vi "motor_controller.vi"() -> ()   [LabVIEW 2015]
uses:
  <vilib>/Analysis/baseanly.llb/Mean (DBL).vi
  <vilib>/Analysis/NI_AALBase.lvlib
panel:
  out "Grapher VI":refnum<vi>
  out "Simulation VI":refnum<vi>
  in  "Make up fit parameters":bool
  in  "Automatic velocity (rev/sec)":dbl=0.1 min=0.0 max=1.0
  in  "Reseek":bool
  in  "Automatic step size (rev)":dbl=0.01 min=0.0 max=1.0
  in  "Refine fit parameters":bool
  out "Fit parameters":cluster{"Slope":dbl, "Intercept":dbl}
  in  "Calculate fit parameters":bool
  in  "Read position 2":bool
  in  "Read position 1":bool
  out "Position 2":dbl
  in  "Frequency 2":dbl=140.4 min=0.0 step=0.001 format="%.3g"
  out "Position 1":dbl
  in  "Frequency 1":dbl=140.0 min=0.0 step=0.001 format="%.3g"
  in  "Seek positive polarization":bool=TRUE
  in  "Launch simulation":bool
  out "Polarization":dbl
  out "Eventnum":i64
  out "Samples taken":i32
  out "Rate":dbl
  in  "Data input file":path
  in  "Automatic mode on/off":bool
  in  "Goto frequency":bool
  in  "Frequency to seek (GHz)":dbl format="%.3g"
  in  "Stop motor":bool
  in  "Move up":bool
  in  "Move down":bool
  in  "Velocity (rev/sec)":dbl min=0.0 max=1.0 step=0.001
  in  "Step size (rev)":dbl=0.01 min=0.0 max=5.0 step=0.001
  in  "Stop communication":bool
  in  "COM Port":refnum<visa-resource-name>
  out "Alarm":bool
  out "Alarm code":u32 format="0x%02x"
  out "Frequency (calculated, GHz)":dbl format="%.3g"
  out "Motor position (rev)":dbl
  out "Motor time (sec)":dbl
  # "Advanced configuration"
  # "Frequency calibration"
  # "Automatic control"
  # "Manual motor control"
  # "Communication setup"
  # "Please wait after stopping the VI; it can take some time to shut down all the stuff running in the background, so please be patient."
  # "Motor alarm (error)"
  # "See motor manual, section \"Troubleshooting\" for explanation of alarm codes; fix the problem first and then restart this VI"
  # "Motor information"
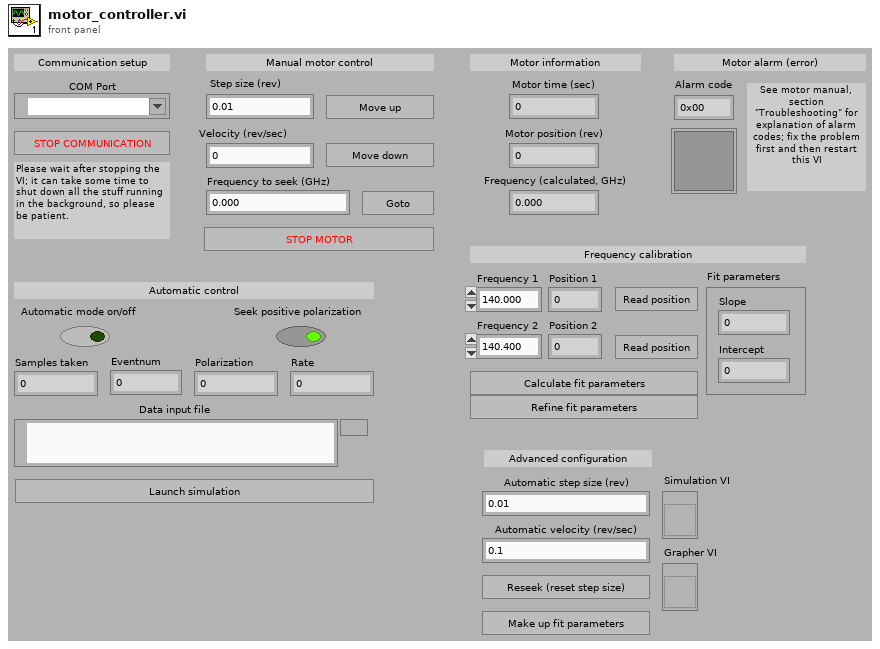
[diagram p1: front panel]
types:
  T1 = typedef "Semaphore RefNum" = refnum<k1>
  T2 = enum8{"Enabled", "Disabled", "Disabled and Grayed Out"}
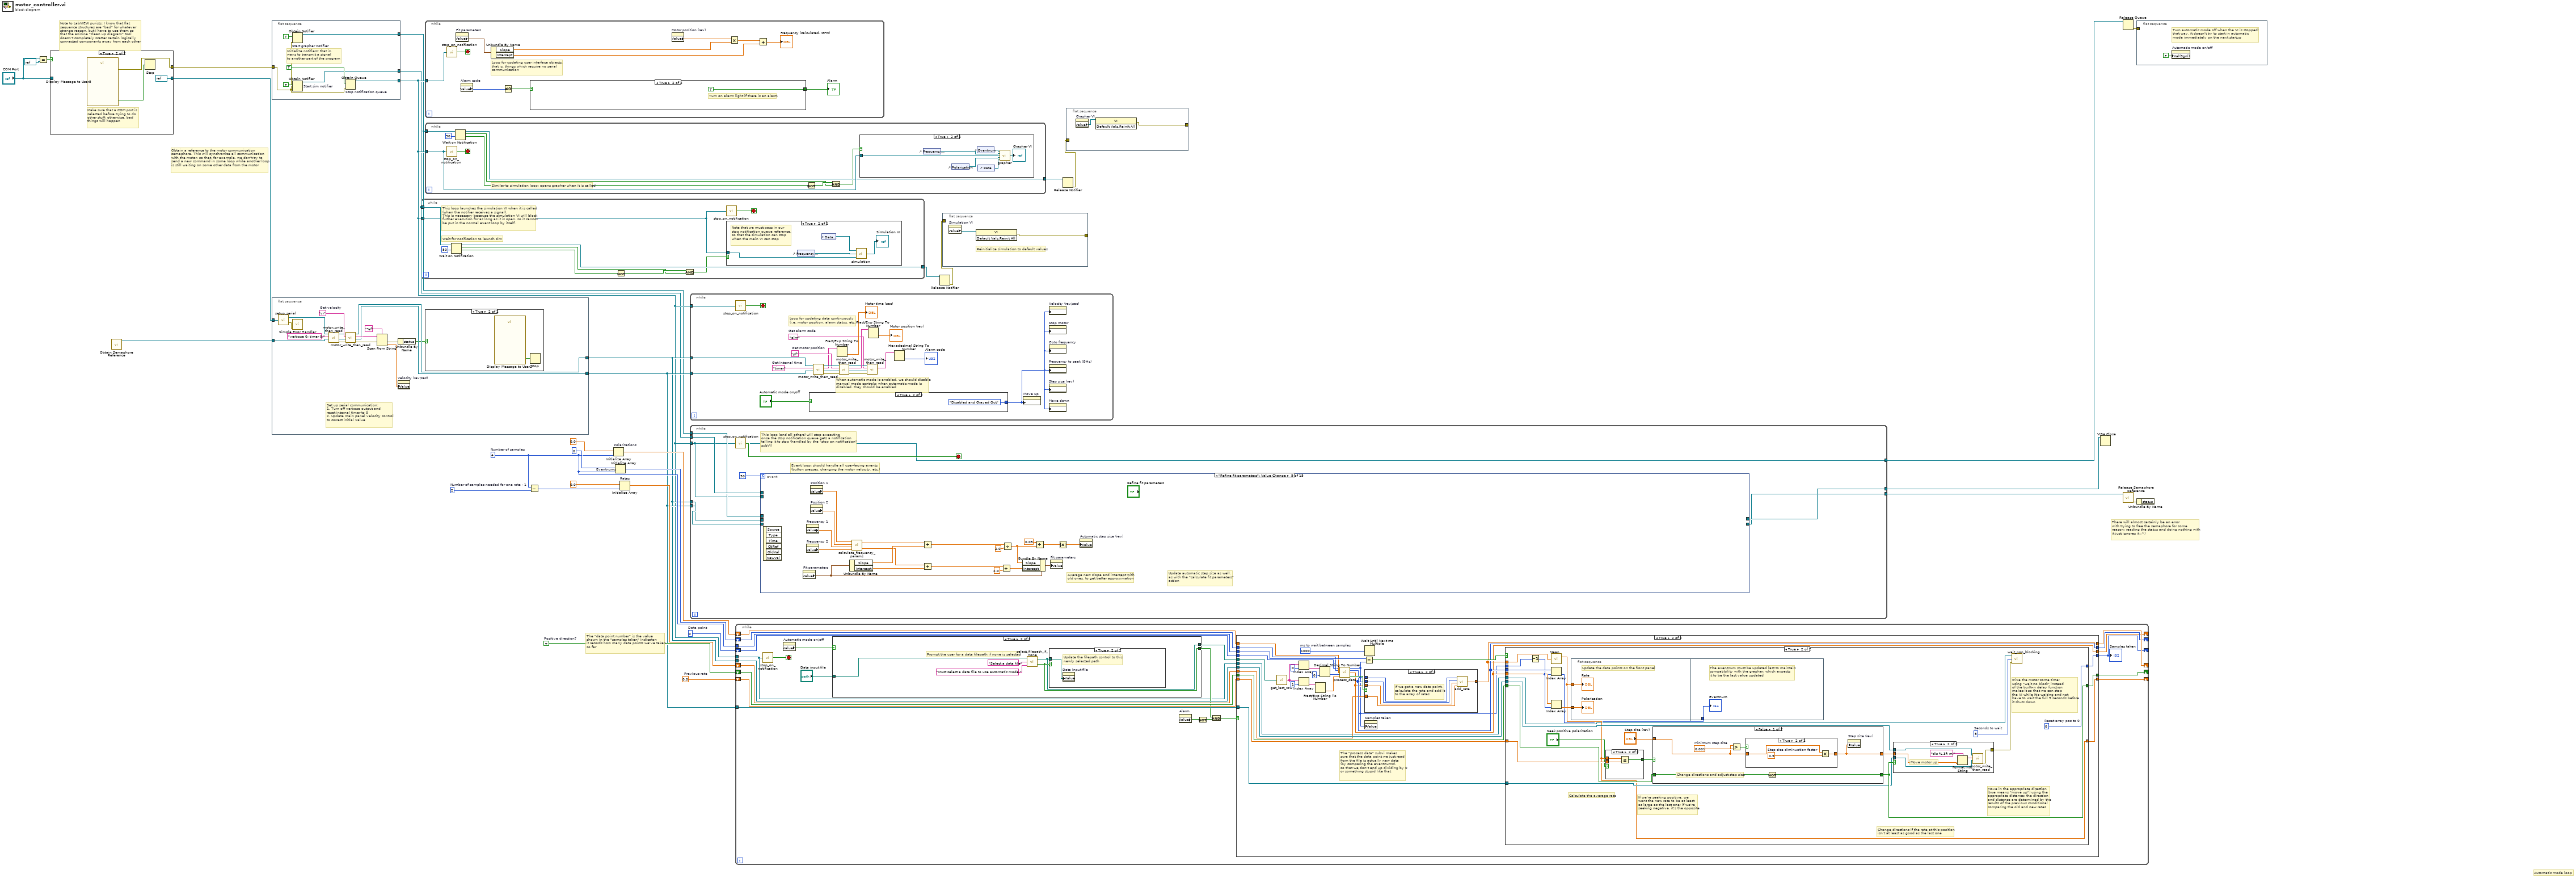
[diagram p0: block diagram]
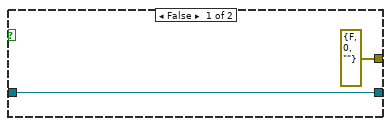
[diagram p4: hidden frame]
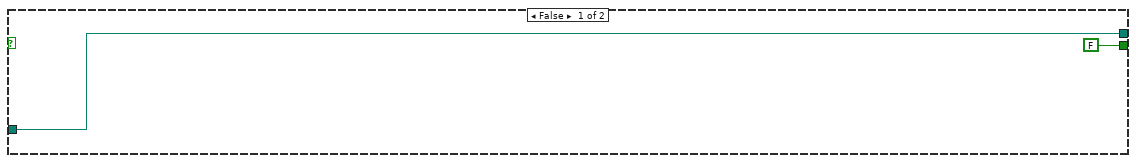
[diagram p6: hidden frame]
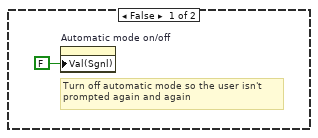
[diagram p7: hidden frame]
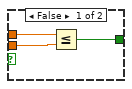
[diagram p11: hidden frame]
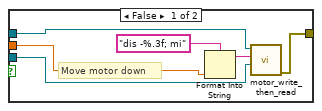
[diagram p12: hidden frame]
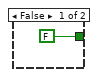
[diagram p15: hidden frame]
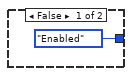
[diagram p16: hidden frame]
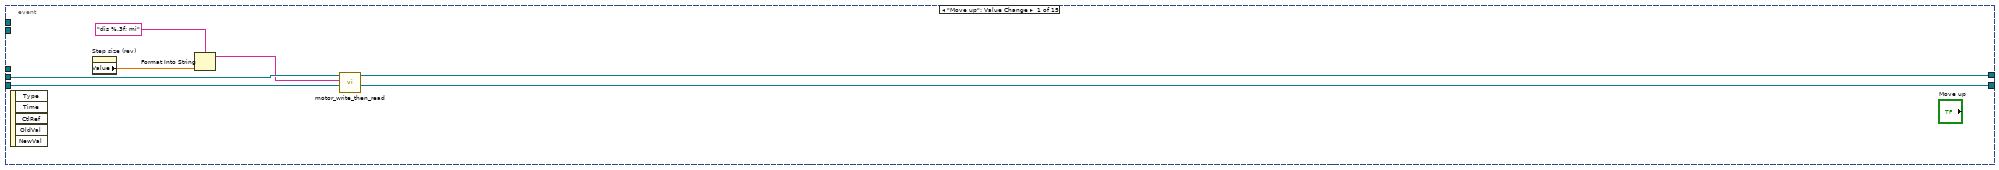
[diagram p17: hidden frame]
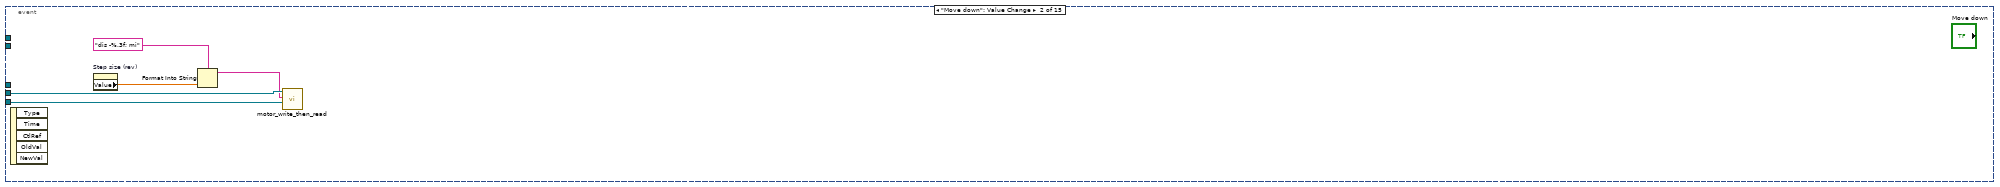
[diagram p18: hidden frame]
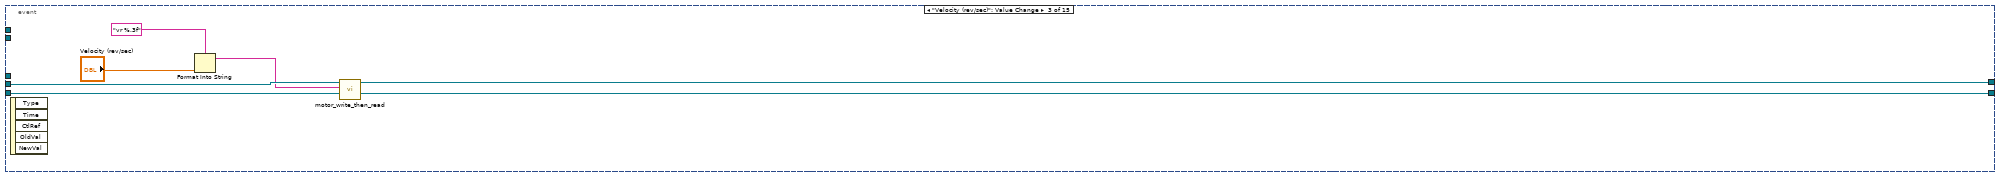
[diagram p19: hidden frame]
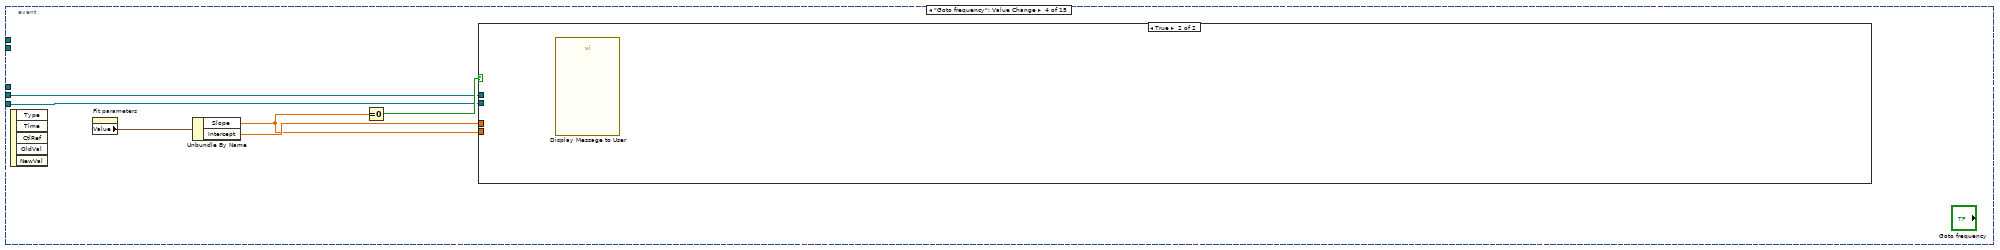
[diagram p20: hidden frame]
diagram:
  w17 = TRUE  # Positive direction?
  w18 = 0.0  # Previous rate
  w21 = 2  # Number of samples needed for one rate - 1
  w19 = 4  # Number of samples
  w28 = 0  # Data point
  # "There will almost certainly be an error\nwith trying to free the semaphore for some\nreason; reading the status and doing nothing with\nit just ignores it :^)"
  # "Obtain a reference to the motor communication\nsemaphore. This will synchronize all communication\nwith the motor, so that, for example, we don't try to\nsend a new command in some loop while another loop\nis still waiting on some other data from the motor"
  # "The \"data point number\" is the value\nshown in the \"samples taken\" indicator;\nit records how many data points we've taken\nso far"
  # "Automatic mode loop"
  # "Note to LabVIEW purists: I know that flat\nsequence structures are \"bad\" for whatever\nstrange reason, but I have to use them so\nthat the asinine \"clean up diagram\" tool\ndoesn't completely scatter certain logically\nconnected components away from each other"
  n1 = Equal?(x="COM Port", y=refnum<visa-resource-name> refnum) -> (x = y?=w12:bool)
  n2 = case shown="True" w12 {
    tunnel: "COM Port" -> [w34 _]
    tunnel: [w34 refnum<visa-resource-name> refnum ("COM Port")] -> w8
    tunnel: [errorcluster {"status"=FALSE, "code"=0, "source"=""} ("error out") w35] -> w3
    frame False {
    }
    frame True {
      # "Make sure that a COM port is\nselected before trying to do\nother stuff; otherwise, bad\nthings will happen"
      n3 = call "Display Message to User5"() -> ("error out"=w35:errorcluster, "I'm very sorry"=w36:bool)  [unwired: 10 in]
      n4 = Stop(stop? (T)=w36) -> ()
    }
  }
  n5 = call <vilib>:"Obtain Semaphore Reference.vi"() -> ("semaphore"=w7:T1)  [unwired: 5 in, 2 out]
  n6 = flat-sequence {
    tunnel: [w41] -> w6
    tunnel: [w40] -> w5
    tunnel: [w39] -> w4
    tunnel: w3 -> [w38]
    frame #0 {
      # "Initialize notifiers; that is,\nways to transmit a signal\nto another part of the program"
      n7 = Obtain Notifier "Start grapher notifier"(notification data type=TRUE, error in (no error)=w38) -> (notifier out=w40:refnum<notifier>)  [unwired: 2 in, 2 out]
      n8 = Obtain Notifier "Start sim notifier"(notification data type=TRUE, error in (no error)=w38) -> (notifier out=w39:refnum<notifier>)  [unwired: 2 in, 2 out]
      n9 = Obtain Queue "Stop notification queue"(element data type=TRUE, error in (no error)=w38) -> (queue out=w41:refnum<queue>)  [unwired: 3 in, 2 out]
    }
  }
  n10 = flat-sequence {
    tunnel: [w48] -> w10
    tunnel: [w49] -> w9
    tunnel: w8 -> [w50]
    tunnel: w7 -> [w47]
    frame #0 {
      w58 = "vr"  # Get velocity
      # "Set up serial communication:\n1. Turn off verbose output and\nreset internal timer to 0\n2. Update main panel velocity control\nto correct initial value"
      n11 = call "setup_serial.vi"("COM Port"=w50) -> ("error out"=w52:errorcluster, "VISA resource name out"=w55:refnum<visa-resource-name>)
      n12 = call <vilib>:"Simple Error Handler.vi"("error in (no error)"=w52) -> ()  [unwired: 4 in, 5 out]
      n13 = call "motor_write_then_read.vi"("Semaphore in"=w47, "Data to write"="verbose 0; timer 0;", "VISA resource name in"=w55) -> ("Error out"=w61:errorcluster, "Semaphore out"=w51:T1, "VISA resource name out"=w57:refnum<visa-resource-name>)  [unwired: 1 in, 1 out]
      n14 = call "motor_write_then_read.vi"("Error in"=w61, "Semaphore in"=w51, "Data to write"=w58, "VISA resource name in"=w57) -> ("Error out"=w60:errorcluster, "Semaphore out"=w48:T1, "Received data"=w59:string, "VISA resource name out"=w49:refnum<visa-resource-name>)
      n15 = Scan From String(format string="%f", input string=w59, error in=w60) -> (error out=w46:errorcluster, output 1=w54:dbl)  [unwired: 2 in, 2 out]
      n16 = Unbundle By Name(w46) -> ("status"=w45:bool)
      n17 = property on="Velocity (rev/sec)" class="DigNum (strict)"("Value"=w54) -> ()  [unwired: 2 in, 2 out]
      n18 = case shown="True" w45 {
        frame False {
        }
        frame True {
          n19 = call "Display Message to User2"() -> ("Thanks, I'll try that"=w62:bool)  [unwired: 10 in, 1 out]
          n20 = Stop(stop? (T)=w62) -> ()
        }
      }
    }
  }
  n21 = while {
    tunnel: w6 -> [w63]
    tunnel: w4 -> [w69]
    tunnel: [w68] -> w15
    stop <- w71 stop-if-true
    # "This loop launches the simulation VI when it is called\n(when the notifier receives a signal).\nThis is necessary because the simulation VI will block\nfurther execution for as long as it is open, so it cannot\nbe put in the normal event loop by itself."
    # "Wait for notification to launch sim"
    n22 = Wait on Notification(notifier=w69, timeout in ms (-1)=50) -> (notifier out=w68:refnum<notifier>, notification=w65:bool, timed out?=w66:bool)  [unwired: 2 in, 1 out]
    n23 = Not(x=w66) -> (.not. x?=w67:bool)
    n24 = And(x=w67, y=w65) -> (x .and. y?=w64:bool)
    n25 = call "stop_on_notification.vi"("Notofication queue"=w63) -> ("Should stop"=w71:bool)
    n26 = case shown="True" w64 {
      tunnel: w63 -> [_ w75]
      frame False {
      }
      frame True {
        # "Note that we must pass in our\nstop notification queue reference,\nso that the simulation can stop\nwhen the main VI can stop"
        n27 = control-ref of="Frequency (calculated, GHz)"() -> (w74:refnum<vi>)
        n28 = control-ref of="Data input file"() -> (w73:refnum<vi>)
        n29 = call "simulation.vi"("Stop notification queue"=w75, "Frequency refnum"=w74, "Filepath refnum"=w73) -> ("This VI refnum"=→"Simulation VI":refnum<vi>)
      }
    }
  }
  n30 = while {
    tunnel: w6 -> [w79]
    stop <- w78 stop-if-true
    # "Loop for updating user interface objects,\nthat is, things which require no serial\ncommunication"
    n31 = call "stop_on_notification.vi"("Notofication queue"=w79) -> ("Should stop"=w78:bool)
    n32 = property on="Fit parameters" class="Clust (strict)"() -> ("Value"=w85:cluster{"Slope":dbl, "Intercept":dbl})  [unwired: 2 in, 2 out]
    n33 = property on="Alarm code" class="DigNum (strict)"() -> ("Value"=w77:u32)  [unwired: 2 in, 2 out]
    n34 = Unbundle By Name(w85) -> ("Slope"=w83:dbl, "Intercept"=w80:dbl)
    n35 = Not Equal To 0?(x=w77) -> (x != 0?=w76:bool)
    n36 = case shown="True" w76 {
      tunnel: [FALSE TRUE] -> w86
      frame False {
      }
      frame True {
        # "Turn on alarm light if there is an alarm"
      }
    }
    "Alarm" <- w86
    n37 = property on="Motor position (rev)" class="DigNum (strict)"() -> ("Value"=w84:dbl)  [unwired: 2 in, 2 out]
    n38 = Multiply(x=w84, y=w83) -> (x*y=w81:dbl)
    n39 = Add(x=w81, y=w80) -> (x+y=→"Frequency (calculated, GHz)":dbl)
  }
  n40 = while {
    tunnel: w6 -> [w96]
    tunnel: w5 -> [w94]
    tunnel: [w93] -> w11
    stop <- w97 stop-if-true
    # "Similar to simulation loop; opens grapher when it is called"
    n41 = call "stop_on_notification.vi"("Notofication queue"=w96) -> ("Should stop"=w97:bool)
    n42 = Wait on Notification(notifier=w94, timeout in ms (-1)=50) -> (notifier out=w93:refnum<notifier>, notification=w91:bool, timed out?=w90:bool)  [unwired: 2 in, 1 out]
    n43 = Not(x=w90) -> (.not. x?=w92:bool)
    n44 = And(x=w92, y=w91) -> (x .and. y?=w89:bool)
    n45 = case shown="True" w89 {
      tunnel: w96 -> [_ w100]
      frame False {
      }
      frame True {
        n46 = control-ref of="Frequency (calculated, GHz)"() -> (w101:refnum<vi>)
        n47 = control-ref of="Polarization"() -> (w102:refnum<vi>)
        n48 = control-ref of="Eventnum"() -> (w99:refnum<vi>)
        n49 = control-ref of="Rate"() -> (w103:refnum<vi>)
        n50 = call "grapher.vi"("Eventnum refnum"=w99, "Frequency refnum"=w101, "Stop notification queue"=w100, "Polarization refnum"=w102, "Rate refnum"=w103) -> ("This VI refnum"=→"Grapher VI":refnum<vi>)  [unwired: 10 in]
      }
    }
  }
  n51 = Subtract(x=w19, y=w21) -> (x-y=w22:i32)
  n52 = Initialize Array "Polarizations"(0.0, w19) -> (w25:dbl[])
  n53 = Initialize Array "Eventnums"(i64 0, w19) -> (w26:i64[])
  n54 = Initialize Array "Rates"(0.0 ("element"), w22) -> (w20:dbl[])
  n55 = while {
    tunnel: w10 -> [w123]
    tunnel: w9 -> [w124]
    tunnel: w6 -> [w106]
    stop <- w105 stop-if-true
    w110 = "alm"  # Get alarm code
    w118 = "pf"  # Get motor position
    w122 = "timer"  # Get internal time
    # "When automatic mode is enabled, we should disable\nmanual mode controls; when automatic mode is\ndisabled, they should be enabled"
    # "Loop for updating data continuously\n(i.e. motor position, alarm status, etc.)"
    n56 = call "stop_on_notification.vi"("Notofication queue"=w106) -> ("Should stop"=w105:bool)
    n57 = case shown="True" "Automatic mode on/off" {
      tunnel: [T2."Enabled" ("Disabled") T2."Disabled and Grayed Out" ("Disabled")] -> w104
      frame False {
      }
      frame True {
      }
    }
    n58 = call "motor_write_then_read.vi"("Semaphore in"=w123, "Data to write"=w122, "VISA resource name in"=w124) -> ("Error out"=w119:errorcluster, "Semaphore out"=w120:T1, "Received data"=w117:string, "VISA resource name out"=w121:refnum<visa-resource-name>)  [unwired: 1 in]
    n59 = Fract/Exp String To Number(string=w117) -> (number=→"Motor time (sec)":dbl)  [unwired: 3 in, 1 out]
    n60 = call "motor_write_then_read.vi"("Error in"=w119, "Semaphore in"=w120, "Data to write"=w118, "VISA resource name in"=w121) -> ("Error out"=w112:errorcluster, "Semaphore out"=w111:T1, "Received data"=w115:string, "VISA resource name out"=w113:refnum<visa-resource-name>)
    n61 = call "motor_write_then_read.vi"("Error in"=w112, "Semaphore in"=w111, "Data to write"=w110, "VISA resource name in"=w113) -> ("Received data"=w109:string)  [unwired: 3 out]
    n62 = Fract/Exp String To Number(string=w115) -> (number=→"Motor position (rev)":dbl)  [unwired: 3 in, 1 out]
    n63 = Hexadecimal String To Number(string=w109) -> (number=→"Alarm code":u32)  [unwired: 2 in, 1 out]
    n64 = property on="Move up" class="Bool"("DisabledEnum"=w104) -> ()  [unwired: 2 in, 2 out]
    n65 = property on="Velocity (rev/sec)" class="DigNum (strict)"("DisabledEnum"=w104) -> ()  [unwired: 2 in, 2 out]
    n66 = property on="Stop motor" class="Bool"("DisabledEnum"=w104) -> ()  [unwired: 2 in, 2 out]
    n67 = property on="Goto frequency" class="Bool"("DisabledEnum"=w104) -> ()  [unwired: 2 in, 2 out]
    n68 = property on="Frequency to seek (GHz)" class="DigNum (strict)"("DisabledEnum"=w104) -> ()  [unwired: 2 in, 2 out]
    n69 = property on="Step size (rev)" class="DigNum (strict)"("DisabledEnum"=w104) -> ()  [unwired: 2 in, 2 out]
    n70 = property on="Move down" class="Bool"("DisabledEnum"=w104) -> ()  [unwired: 2 in, 2 out]
  }
  n71 = while {
    tunnel: w10 -> [w135]
    tunnel: w9 -> [w134]
    tunnel: [w133] -> w32
    tunnel: [w132] -> w31
    tunnel: w6 -> [w127]
    tunnel: [w127] -> w29
    tunnel: w4 -> [w131]
    tunnel: w5 -> [w130]
    stop <- w129 stop-if-true
    # "This loop (and all others) will stop executing\nonce the stop notification queue gets a notification\ntelling it to stop (handled by the \"stop on notification\"\nsubVI)"
    # "Event loop; should handle all user-facing events\n(button presses, changing the motor velocity, etc.)"
    n72 = call "stop_on_notification.vi"("Notofication queue"=w127) -> ("Should stop"=w129:bool)
    n73 = event shown="[8] \"Refine fit parameters\": Value Change" {
      selector: _ -> [_ _ _ _ _ _ _ _ _ _ _ _ _ _ _]
      dyn-events: _ -> [_ _ _ _ _ _ _ _ _ _ _ _ _ _ _]
      timeout: 50 -> [_ _ _ _ _ _ _ _ _ _ _ _ _ _ _]
      tunnel: w135 -> [w139 w143 w150 w155 w186 _ _ _ _ _ _ _ _ _ w250]
      tunnel: w134 -> [w140 w145 w152 w156 w192 _ _ _ _ _ _ _ _ _ w251]
      tunnel: [w138 _ w148 _ _ _ _ _ _ _ _ _ _ _ w251] -> w133
      tunnel: [w137 _ w149 _ _ _ _ _ _ _ _ _ _ _ w250] -> w132
      tunnel: w131 -> [_ _ _ _ _ _ _ _ _ w228 _ _ _ _ _]
      tunnel: w130 -> [_ _ _ _ _ _ _ _ _ _ _ w236 _ _ _]
      tunnel: w127 -> [_ _ _ _ _ _ _ _ _ _ _ _ _ w248 _]
      event "Move up": Value Change {
        n74 = event-data() -> ()  [unwired: 1 in, 5 out]
        n75 = property on="Step size (rev)" class="DigNum (strict)"() -> ("Value"=w141:dbl)  [unwired: 2 in, 2 out]
        n76 = Format Into String(format string="dis %.3f; mi", w141) -> (resulting string=w136:string)  [unwired: 2 in, 1 out]
        n77 = call "motor_write_then_read.vi"("Semaphore in"=w139, "Data to write"=w136, "VISA resource name in"=w140) -> ("Semaphore out"=w137:T1, "VISA resource name out"=w138:refnum<visa-resource-name>)  [unwired: 1 in, 2 out]
      }
      event "Move down": Value Change {
        n78 = event-data() -> ()  [unwired: 1 in, 5 out]
        n79 = property on="Step size (rev)" class="DigNum (strict)"() -> ("Value"=w146:dbl)  [unwired: 2 in, 2 out]
        n80 = Format Into String(format string="dis -%.3f; mi", w146) -> (resulting string=w144:string)  [unwired: 2 in, 1 out]
        n81 = call "motor_write_then_read.vi"("Semaphore in"=w143, "Data to write"=w144, "VISA resource name in"=w145) -> ()  [unwired: 1 in, 4 out]
      }
      event "Velocity (rev/sec)": Value Change {
        n82 = event-data() -> ()  [unwired: 1 in, 5 out]
        n83 = Format Into String(format string="vr %.3f", "Velocity (rev/sec)") -> (resulting string=w151:string)  [unwired: 2 in, 1 out]
        n84 = call "motor_write_then_read.vi"("Semaphore in"=w150, "Data to write"=w151, "VISA resource name in"=w152) -> ("Semaphore out"=w149:T1, "VISA resource name out"=w148:refnum<visa-resource-name>)  [unwired: 1 in, 2 out]
      }
      event "Goto frequency": Value Change {
        n85 = event-data() -> ()  [unwired: 1 in, 5 out]
        n86 = property on="Fit parameters" class="Clust (strict)"() -> ("Value"=w160:cluster{"Slope":dbl, "Intercept":dbl})  [unwired: 2 in, 2 out]
        n87 = Unbundle By Name(w160) -> ("Slope"=w157:dbl, "Intercept"=w158:dbl)
        n88 = Equal To 0?(x=w157) -> (x = 0?=w159:bool)
        n89 = case shown="True" w159 {
          tunnel: w158 -> [w173 _]
          tunnel: w157 -> [w171 _]
          tunnel: w156 -> [w168 _]
          tunnel: w155 -> [w167 _]
          frame False {
            # "Calculate corresponding motor position and go there"
            n90 = Subtract(x="Frequency to seek (GHz)", y=w173) -> (x-y=w172:dbl)
            n91 = property on="Motor position (rev)" class="DigNum (strict)"() -> ("Value"=w169:dbl)  [unwired: 2 in, 2 out]
            n92 = Divide(x=w172, y=w171) -> (x/y=w170:dbl)
            n93 = Subtract(x=w170, y=w169) -> (x-y=w165:dbl)
            n94 = Absolute Value(x=w165) -> (abs(x)=w164:dbl)
            n95 = Less?(x=w164, y=1.0) -> (x < y?=w161:bool)
            n96 = case shown="False" w161 {
              selector: w161 -> [_ w178]
              tunnel: [w174 w178] -> w162
              frame False {
                n97 = Two Button Dialog(message="The frequency you are attempting to go to is very far from the current position; you may run into problems. Are you sure you want to continue?", 1:"No" ("F button name (\"Cancel\")"), 2:"Yes" ("T button name (\"OK\")")) -> (T button?=w174:bool)
              }
              frame True {
              }
            }
            n98 = case shown="True" w162 {
              tunnel: w168 -> [_ w183]
              tunnel: w165 -> [_ w182]
              tunnel: w167 -> [_ w179]
              frame False {
              }
              frame True {
                n99 = Format Into String(format string="dis %.3f; mi", w182) -> (resulting string=w180:string)  [unwired: 2 in, 1 out]
                n100 = call "motor_write_then_read.vi"("Semaphore in"=w179, "Data to write"=w180, "VISA resource name in"=w183) -> ()  [unwired: 1 in, 4 out]
              }
            }
          }
          frame True {
            n101 = call "Display Message to User"() -> ()  [unwired: 10 in, 2 out]
          }
        }
      }
      event "Stop motor": Value Change {
        n102 = event-data() -> ()  [unwired: 1 in, 5 out]
        n103 = call <vilib>:"Acquire Semaphore.vi"("semaphore"=w186) -> ("error out"=w190:errorcluster, "semaphore out"=w185:T1)  [unwired: 4 in, 1 out]
        n104 = VISA Write(VISA resource name=w192, write buffer="mstop\r", error in (no error)=w190) -> (VISA resource name out=w194:refnum<visa-resource-name>, error out=w189:errorcluster)  [unwired: 1 out]
        n105 = VISA Read(VISA resource name=w194, byte count=u32 1, error in (no error)=w189) -> (VISA resource name out=w193:refnum<visa-resource-name>, error out=w188:errorcluster)  [unwired: 2 out]
        n106 = VISA Flush I/O Buffer(VISA resource name=w193, error in (no error)=w188) -> (error out=w187:errorcluster)  [unwired: 1 in, 1 out]
        n107 = call <vilib>:"Release Semaphore.vi"("error in (no error)"=w187, "semaphore"=w185) -> ()  [unwired: 4 in, 2 out]
      }
      event "Read position 1": Value Change {
        n108 = event-data() -> ()  [unwired: 1 in, 5 out]
        n109 = property on="Motor position (rev)" class="DigNum (strict)"() -> ("Value"=→"Position 1":dbl)  [unwired: 2 in, 2 out]
      }
      event "Read position 2": Value Change {
        n110 = event-data() -> ()  [unwired: 1 in, 5 out]
        n111 = property on="Motor position (rev)" class="DigNum (strict)"() -> ("Value"=→"Position 2":dbl)  [unwired: 2 in, 2 out]
      }
      event "Calculate fit parameters": Value Change {
        # "The automatic step size should be around 0.05GHz\ninitially, to get a good seek"
        # "Calculate slope and intercept"
        n112 = event-data() -> ()  [unwired: 1 in, 5 out]
        n113 = property on="Position 1" class="DigNum (strict)"() -> ("Value"=w205:dbl)  [unwired: 2 in, 2 out]
        n114 = property on="Position 2" class="DigNum (strict)"() -> ("Value"=w204:dbl)  [unwired: 2 in, 2 out]
        n115 = property on="Calculate fit parameters" class="Bool (strict)"("Value"=FALSE ("Calculate fit parameters")) -> ()  [unwired: 2 in, 2 out]
        n116 = call "calculate_frequency_params.vi"("Frequency 2"="Frequency 2", "Frequency 1"="Frequency 1", "Position 2"=w204, "Position 1"=w205) -> ("Intercept"=w206:dbl, "Slope"=w199:dbl)
        n117 = Divide(x=0.05, y=w199) -> (x/y=w198:dbl)
        n118 = property on="Fit parameters" class="Clust (strict)"() -> ("Value"=w208:cluster{"Slope":dbl, "Intercept":dbl})  [unwired: 2 in, 2 out]
        n119 = Bundle By Name(cluster=w208, "Slope"=w199, "Intercept"=w206) -> (→"Fit parameters":cluster{"Slope":dbl, "Intercept":dbl})
        n120 = Absolute Value(x=w198) -> (abs(x)=w197:dbl)
        n121 = property on="Automatic step size (rev)" class="DigNum (strict)"("Value"=w197) -> ()  [unwired: 2 in, 2 out]
      }
      event "Refine fit parameters": Value Change {
        # "Update automatic step size as well,\nas with the \"calculate fit parameters\"\naction"
        # "Average new slope and intercept with\nold ones, to get better approximation"
        n122 = event-data() -> ()  [unwired: 1 in, 6 out]
        n123 = property on="Fit parameters" class="Clust (strict)"() -> ("Value"=w214:cluster{"Slope":dbl, "Intercept":dbl})  [unwired: 2 in, 2 out]
        n124 = property on="Frequency 1" class="DigNum (strict)"() -> ("Value"=w227:dbl)  [unwired: 2 in, 2 out]
        n125 = property on="Frequency 2" class="DigNum (strict)"() -> ("Value"=w226:dbl)  [unwired: 2 in, 2 out]
        n126 = property on="Position 1" class="DigNum (strict)"() -> ("Value"=w225:dbl)  [unwired: 2 in, 2 out]
        n127 = property on="Position 2" class="DigNum (strict)"() -> ("Value"=w224:dbl)  [unwired: 2 in, 2 out]
        n128 = Unbundle By Name(w214) -> ("Slope"=w222:dbl, "Intercept"=w220:dbl)
        n129 = call "calculate_frequency_params.vi"("Frequency 2"=w226, "Frequency 1"=w227, "Position 2"=w224, "Position 1"=w225) -> ("Intercept"=w221:dbl, "Slope"=w223:dbl)
        n130 = Add(x=w223, y=w222) -> (x+y=w219:dbl)
        n131 = Add(x=w221, y=w220) -> (x+y=w218:dbl)
        n132 = Divide(x=w218, y=2.0) -> (x/y=w213:dbl)
        n133 = Divide(x=w219, y=2.0) -> (x/y=w211:dbl)
        n134 = Bundle By Name(cluster=w214, "Slope"=w211, "Intercept"=w213) -> (w215:cluster{"Slope":dbl, "Intercept":dbl})
        n135 = Divide(x=0.05, y=w211) -> (x/y=w210:dbl)
        n136 = property on="Fit parameters" class="Clust (strict)"("Value"=w215) -> ()  [unwired: 2 in, 2 out]
        n137 = Absolute Value(x=w210) -> (abs(x)=w209:dbl)
        n138 = property on="Automatic step size (rev)" class="DigNum (strict)"("Value"=w209) -> ()  [unwired: 2 in, 2 out]
      }
      event "Launch simulation": Value Change {
        # "Tell the simulation notifier to launch the simulation"
        n139 = event-data() -> ()  [unwired: 1 in, 5 out]
        n140 = property on="Fit parameters" class="Clust (strict)"() -> ("Value"=w231:cluster{"Slope":dbl, "Intercept":dbl})  [unwired: 2 in, 2 out]
        n141 = Unbundle By Name(w231) -> ("Slope"=w230:dbl)
        n142 = Equal To 0?(x=w230) -> (x = 0?=w229:bool)
        n143 = case shown="True" w229 {
          tunnel: w228 -> [w232 _]
          frame False {
            n144 = Send Notification(notification=TRUE, notifier=w232) -> ()  [unwired: 1 in, 2 out]
          }
          frame True {
            n145 = call "Display Message to User3"() -> ()  [unwired: 10 in, 2 out]
          }
        }
      }
      event "Reseek": Value Change {
        # "Change step size back to the default (initial) automatic step size"
        n146 = event-data() -> ()  [unwired: 1 in, 5 out]
        n147 = property on="Automatic mode on/off" class="Bool (strict)"() -> ("Value"=w234:bool)  [unwired: 2 in, 2 out]
        n148 = case shown="True" w234 {
          frame False {
          }
          frame True {
            n149 = property on="Automatic step size (rev)" class="DigNum (strict)"() -> ("Value"=w235:dbl)  [unwired: 2 in, 2 out]
            n150 = property on="Step size (rev)" class="DigNum (strict)"("Value"=w235) -> ()  [unwired: 2 in, 2 out]
          }
        }
      }
      event "Automatic mode on/off": Value Change {
        # "When automatic mode is first enabled,\nchoose the initial step size and start\ngrapher subvi"
        n151 = event-data() -> ()  [unwired: 1 in, 5 out]
        n152 = property on="Automatic mode on/off" class="Bool (strict)"() -> ("Value"=w237:bool)  [unwired: 2 in, 2 out]
        n153 = case shown="True" w237 {
          tunnel: w236 -> [_ w240]
          frame False {
          }
          frame True {
            n154 = Send Notification(notification=TRUE, notifier=w240) -> ()  [unwired: 1 in, 2 out]
            n155 = property on="Velocity (rev/sec)" class="DigNum (strict)"("Val(Sgnl)"="Automatic velocity (rev/sec)") -> ()  [unwired: 2 in, 2 out]
            n156 = property on="Step size (rev)" class="DigNum (strict)"("Val(Sgnl)"="Automatic step size (rev)") -> ()  [unwired: 2 in, 2 out]
          }
        }
      }
      event "Make up fit parameters": Value Change {
        # "Make up some fit parameters (no physical meaning)\nfor quick testing of automatic mode"
        n157 = event-data() -> ()  [unwired: 1 in, 5 out]
        n158 = flat-sequence {
          frame #0 {
            n159 = property on="Frequency 2" class="DigNum (strict)"("Value"=140.15 ("Frequency 2")) -> ()  [unwired: 2 in, 2 out]
            n160 = property on="Frequency 1" class="DigNum (strict)"("Value"=140.1 ("Frequency 1")) -> ()  [unwired: 2 in, 2 out]
            n161 = property on="Motor position (rev)" class="DigNum (strict)"() -> ("Value"=w246:dbl)  [unwired: 2 in, 2 out]
            n162 = property on="Position 2" class="DigNum (strict)"("Value"=w246) -> ()  [unwired: 2 in, 2 out]
            n163 = property on="Step size (rev)" class="DigNum (strict)"() -> ("Value"=w244:dbl)  [unwired: 2 in, 2 out]
            n164 = Subtract(x=w246, y=w244) -> (x-y=w245:dbl)
            n165 = property on="Position 1" class="DigNum (strict)"("Value"=w245) -> ()  [unwired: 2 in, 2 out]
          }
          frame #1 {
            n166 = property on="Calculate fit parameters" class="Bool (strict)"("Val(Sgnl)"=TRUE ("Value (Signaling)")) -> ()  [unwired: 2 in, 2 out]
          }
        }
      }
      event "Stop communication": Value Change {
        n167 = event-data() -> ()  [unwired: 1 in, 5 out]
        n168 = call "send_notification.vi"("Notification"="Stop communication", "Notification queue in"=w248) -> ()  [unwired: 1 out]
      }
      event Timeout {
        n169 = event-data() -> ()  [unwired: 1 in, 2 out]
      }
    }
  }
  n170 = while {
    tunnel: w6 -> [w252]
    shift-right: [w261] -> _
    shift-left: w28 -> [w257]
    shift-right: [w260] -> _
    shift-left: w26 -> [w271]
    shift-right: [w259] -> _
    shift-left: w25 -> [w270]
    shift-right: [w269] -> _
    shift-left: w20 -> [w262]
    tunnel: w19 -> [w268]
    shift-right: [w258] -> _
    shift-left: w18 -> [w267]
    shift-right: [w265] -> _
    shift-left: w17 -> [w266]
    tunnel: w9 -> [w264]
    tunnel: w10 -> [w263]
    stop <- w275 stop-if-true
    n171 = call "stop_on_notification.vi"("Notofication queue"=w252) -> ("Should stop"=w275:bool)
    n172 = property on="Automatic mode on/off" class="Bool (strict)"() -> ("Value"=w256:bool)  [unwired: 2 in, 2 out]
    n173 = case shown="True" w256 {
      tunnel: "Data input file" -> [w277 w280]
      tunnel: [w277 w278] -> w254
      tunnel: [FALSE ("Filepath valid?") w279] -> w253
      frame False {
      }
      frame True {
        # "Prompt the user for a data filepath if none is selected"
        n174 = call "select_filepath_if_none.vi"("Error message"="Must select a data file to use automatic mode.", "Selector prompt"="Select a data file", "Filepath in"=w280) -> ("Filepath valid?"=w279:bool, "Filepath out"=w278:path)
        n175 = case shown="True" w279 {
          tunnel: w278 -> [_ w284]
          frame False {
            # "Turn off automatic mode so the user isn't\nprompted again and again"
            n176 = property on="Automatic mode on/off" class="Bool (strict)"("Val(Sgnl)"=FALSE ("Value (Signaling)")) -> ()  [unwired: 2 in, 2 out]
          }
          frame True {
            # "Update the filepath control to this\nnewly selected path"
            n177 = property on="Data input file" class="Path"("Value"=w284) -> ()  [unwired: 2 in, 2 out]
          }
        }
      }
    }
    n178 = property on="Alarm" class="Bool (strict)"() -> ("Value"=w274:bool)  [unwired: 2 in, 2 out]
    n179 = Not(x=w274) -> (.not. x?=w273:bool)
    n180 = And(x=w253, y=w273) -> (x .and. y?=w272:bool)
    n181 = case shown="True" w272 {
      tunnel: w257 -> [w290 w294]
      tunnel: w271 -> [w289 w300]
      tunnel: w270 -> [w288 w301]
      tunnel: [w290 w313] -> w261
      tunnel: [w289 w298] -> w260
      tunnel: [w288 w297] -> w259
      tunnel: w262 -> [w287 w296]
      tunnel: [w287 w295] -> w269
      tunnel: w268 -> [_ w315]
      tunnel: [w286 w312] -> w258
      tunnel: w267 -> [w286 w311]
      tunnel: w266 -> [w285 w310]
      tunnel: [w285 w309] -> w265
      tunnel: w264 -> [_ w308]
      tunnel: w263 -> [_ w307]
      tunnel: w254 -> [_ w304]
      tunnel: w252 -> [_ w292]
      frame False {
      }
      frame True {
        w305 = u32 1000  # ms to wait between samples
        # "The \"process data\" subvi makes\nsure that the data point we just read\nfrom the file is actually new data\n(by comparing the eventnums),\nso that we don't end up dividing by 0\nor something stupid like that"
        n182 = call "get_last_row.vi"("Data input file"=w304) -> ("last row"=w306:string[])
        n183 = Index Array(array=w306, index=0) -> (element=w317:string)
        n184 = Index Array(array=w306, index=1) -> (element=w316:string)
        n185 = Fract/Exp String To Number(string=w316) -> (number=w302:dbl)  [unwired: 3 in, 1 out]
        n186 = Decimal String To Number(string=w317, default (0L)=i64 0 ("default (0 I32)")) -> (number=w303:i64)  [unwired: 1 in, 1 out]
        n187 = call "process_data.vi"("Array position in"=w294, "Eventnum array in"=w300, "Polarization array in"=w301, "New eventnum"=w303, "New polarization"=w302) -> ("Array position out"=w291:i32, "Eventnum array out"=w298:i64[], "Polarization array out"=w297:dbl[], "Added data point"=w299:bool)  [unwired: 7 in]
        n188 = Equal?(x=w315, y=w291) -> (x = y?=w314:bool)
        n189 = Wait Until Next ms Multiple(millisecond multiple=w305) -> ()  [unwired: 1 out]
        n190 = case shown="True" w299 {
          tunnel: w291 -> [_ w325]
          tunnel: w298 -> [_ w324]
          tunnel: w297 -> [_ w323]
          tunnel: w296 -> [w320 w322]
          tunnel: [w320 w321] -> w295
          frame False {
            # "If we didn't get a new data point,\ndon't do anything"
          }
          frame True {
            # "If we got a new data point,\ncalculate the rate and add it\nto the array of rates"
            n191 = call "add_rate.vi"("Rate array in"=w322, "Polarization array"=w323, "Eventnum array"=w324, "Array position"=w325) -> ("Rate array out"=w321:dbl[])
          }
        }
        n192 = property on="Samples taken" class="DigNum (strict)"("Value"=w291) -> ()  [unwired: 2 in, 2 out]
        n193 = case shown="True" w314 {
          tunnel: [w326 w349] -> w313
          tunnel: [w328 w339] -> w312
          tunnel: w311 -> [w328 w342]
          tunnel: w310 -> [w327 w348]
          tunnel: [w327 w347] -> w309
          tunnel: w308 -> [_ w346]
          tunnel: w307 -> [_ w345]
          tunnel: w291 -> [w326 w334]
          tunnel: w298 -> [_ w337]
          tunnel: w297 -> [_ w336]
          tunnel: w295 -> [_ w335]
          tunnel: w292 -> [_ w332]
          frame False {
          }
          frame True {
            w330 = 5  # Seconds to wait
            w349 = 0  # Reset array pos to 0
            # "Move in the appropriate direction\n(true means \"move up\") using the\nappropriate distance; the direction\nand distance are determined by the\nresults of the previous conditional\ncomparing the old and new rates"
            # "Change directions if the rate at this position\nisn't at least as good as the last one"
            # "If we're seeking positive, we\nwant the new rate to be at least\nas large as the last one; if we're\nseeking negative, it's the opposite"
            # "Give the motor some time;\nusing \"wait no block\" instead\nof the built-in delay function\nmakes it so that we can stop\nthe VI while it's waiting and not\nhave to wait the full 5 seconds before\nit shuts down"
            # "Calculate the average rate"
            n194 = Decrement(x=w334) -> (x-1=w333:i32)
            n195 = call-poly <vilib>:"Mean.vi"("X"=w335) -> ("mean"=w339:dbl)  [unwired: 1 out]
            n196 = Index Array(array=w337, index=w333) -> (element=w338:i64)
            n197 = Index Array(array=w336, index=w333) -> (element=w340:dbl)
            n198 = flat-sequence {
              tunnel: w340 -> [w356]
              tunnel: w339 -> [w357]
              tunnel: w338 -> [w358]
              frame #0 {
                # "Update the data points on the front panel"
                "Polarization" <- w356
                "Rate" <- w357
              }
              frame #1 {
                # "The eventnum must be updated last to maintain\ncompatibility with the grapher, which expects\nit to be the last value updated"
                "Eventnum" <- w358
              }
            }
            n199 = case shown="True" "Seek positive polarization" {
              tunnel: w342 -> [w351 w355]
              tunnel: [w350 w354] -> w341
              tunnel: w339 -> [w352 w353]
              frame False {
                n200 = Less Or Equal?(x=w352, y=w351) -> (x <= y?=w350:bool)
              }
              frame True {
                n201 = Greater Or Equal?(x=w353, y=w355) -> (x >= y?=w354:bool)
              }
            }
            n202 = case shown="False" w341 {
              tunnel: w348 -> [w376 w382]
              tunnel: [w375 w382] -> w347
              tunnel: "Step size (rev)" -> [w372 w381]
              tunnel: [w371 w381] -> w343
              frame False {
                w374 = 0.001  # Minimum step size
                # "Change directions and adjust step size"
                n203 = Greater?(x=w372, y=w374) -> (0:w373:bool)
                n204 = case shown="True" w373 {
                  tunnel: w372 -> [w377 w379]
                  tunnel: [w377 w378] -> w371
                  frame False {
                  }
                  frame True {
                    w380 = 0.9  # Step size diminuation factor
                    n205 = Multiply(x=w379, y=w380) -> (x*y=w378:dbl)
                  }
                }
                n206 = Not(x=w376) -> (.not. x?=w375:bool)
                n207 = property on="Step size (rev)" class="DigNum (strict)"("Value"=w371) -> ()  [unwired: 2 in, 2 out]
              }
              frame True {
              }
            }
            n208 = case shown="True" w347 {
              tunnel: w346 -> [w363 w370]
              tunnel: w345 -> [w364 w369]
              tunnel: [w362 w368] -> w344
              tunnel: w343 -> [w360 w367]
              frame False {
                # "Move motor down"
                n209 = Format Into String(format string="dis -%.3f; mi", w360) -> (resulting string=w359:string)  [unwired: 2 in, 1 out]
                n210 = call "motor_write_then_read.vi"("Semaphore in"=w364, "Data to write"=w359, "VISA resource name in"=w363) -> ("Error out"=w362:errorcluster)  [unwired: 1 in, 3 out]
              }
              frame True {
                # "Move motor up"
                n211 = Format Into String(format string="dis %.3f; mi", w367) -> (resulting string=w365:string)  [unwired: 2 in, 1 out]
                n212 = call "motor_write_then_read.vi"("Semaphore in"=w369, "Data to write"=w365, "VISA resource name in"=w370) -> ("Error out"=w368:errorcluster)  [unwired: 1 in, 3 out]
              }
            }
            n213 = call "wait_non_blocking.vi"("Error in"=w344, "Seconds to wait"=w330, "Stop notification queue"=w332) -> ()
          }
        }
      }
    }
    "Samples taken" <- w261
  }
  n214 = Release Notifier(notifier=w15) -> (error out=w2:errorcluster)  [unwired: 2 in, 2 out]
  n215 = flat-sequence {
    tunnel: w2 -> [_]
    tunnel: [w383] -> _
    frame #0 {
      # "Reinitialize simulation to default values"
      n216 = property on="Simulation VI" class="VIRef (strict)"() -> ("Value"=w384:refnum<vi>)  [unwired: 2 in, 2 out]
      n217 = invoke class="VI" method="Default Vals.Reinit All"(reference=w384) -> (error out=w383:errorcluster)  [unwired: 2 in, 2 out]
    }
  }
  n218 = Release Notifier(notifier=w11) -> (error out=w1:errorcluster)  [unwired: 2 in, 2 out]
  n219 = flat-sequence {
    tunnel: w1 -> [_]
    tunnel: [w385] -> _
    frame #0 {
      n220 = property on="Grapher VI" class="VIRef (strict)"() -> ("Value"=w386:refnum<vi>)  [unwired: 2 in, 2 out]
      n221 = invoke class="VI" method="Default Vals.Reinit All"(reference=w386) -> (error out=w385:errorcluster)  [unwired: 2 in, 2 out]
    }
  }
  n222 = VISA Close(VISA resource name=w32) -> ()  [unwired: 1 in, 1 out]
  n223 = Release Queue(queue=w29) -> (error out=w16:errorcluster)  [unwired: 2 in, 2 out]
  n224 = call <vilib>:"Release Semaphore Reference.vi"("semaphore"=w31) -> ("error out"=w30:errorcluster)  [unwired: 9 in, 1 out]
  n225 = flat-sequence {
    tunnel: w16 -> [_]
    frame #0 {
      # "Turn automatic mode off when the VI is stopped;\nthat way, it doesn't try to start in automatic\nmode immediately on the next startup"
      n226 = property on="Automatic mode on/off" class="Bool (strict)"("Val(Sgnl)"=FALSE ("Automatic mode on/off")) -> ()  [unwired: 2 in, 2 out]
    }
  }
  n227 = Unbundle By Name(w30) -> ()  [unwired: 1 out]
